vi "Set AO Chan Gain on Fly.vi"(8 "error in (no error)":errorcluster, 9 "Gain Setting":u16(ring) items=["0 dB Gain"=0, "20 dB Gain"=2, "40 dB Gain"=4], 10 "channel":string="AO01") -> (0 "error out":errorcluster)   [LabVIEW 2015]
uses:
  PXI Globals.vi
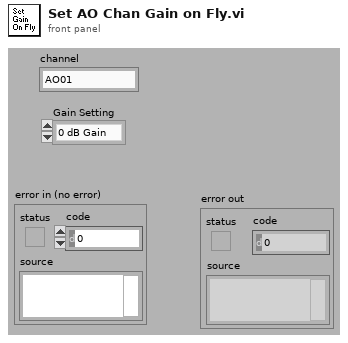
[diagram p1: front panel]
types:
  T1 = typedef "Task Struct.ctl" = cluster{"Task name":string, "Task":refnum<k21>, "Dual-channel task?":bool, "Regenerate?":bool, "Clear?":bool}
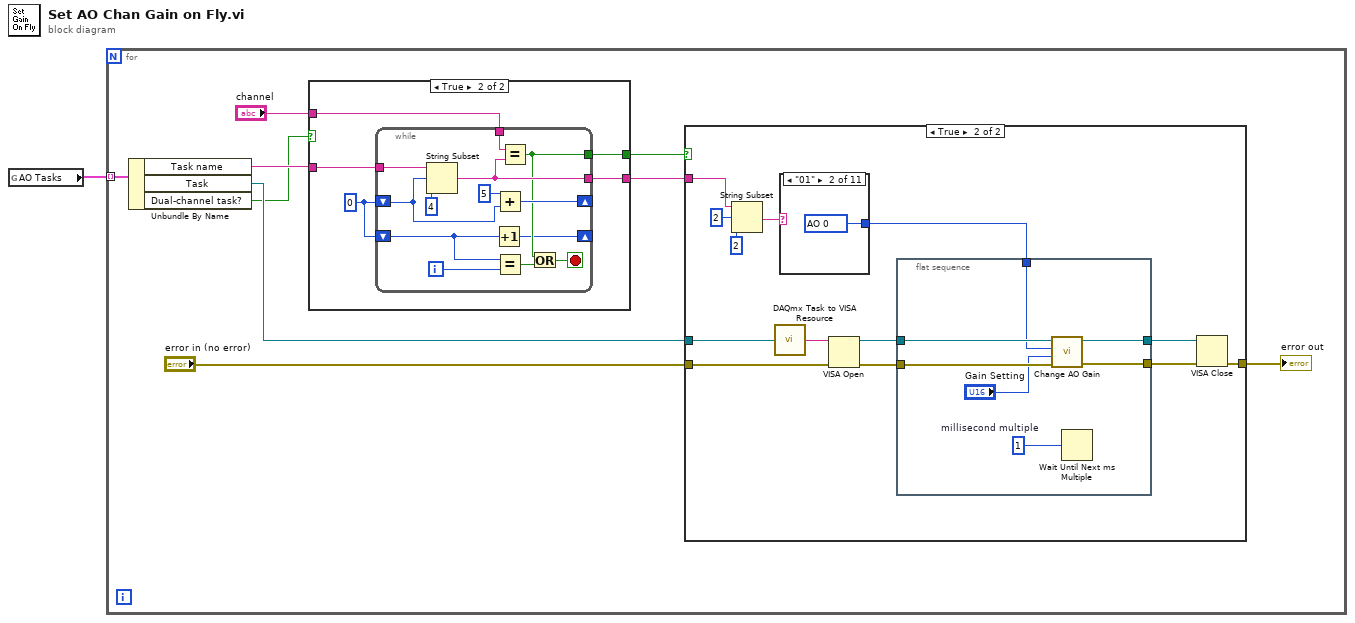
[diagram p0: block diagram]
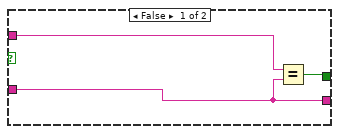
[diagram p2: hidden frame]
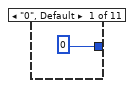
[diagram p4: hidden frame]
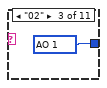
[diagram p5: hidden frame]
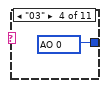
[diagram p6: hidden frame]
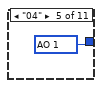
[diagram p7: hidden frame]
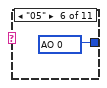
[diagram p8: hidden frame]
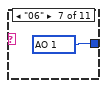
[diagram p9: hidden frame]
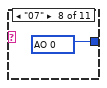
[diagram p10: hidden frame]
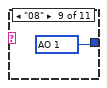
[diagram p11: hidden frame]
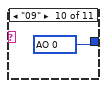
[diagram p12: hidden frame]
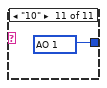
[diagram p13: hidden frame]
diagram:
  n1 = global read "PXI Globals.vi" "AO Tasks"() -> (w1:T1[])
  n2 = for {
    tunnel: w1 -> [w10] mode=indexing
    n3 = Unbundle By Name(w10) -> ("Task name"=w6:string, "Task"=w7:refnum<k21>, "Dual-channel task?"=w5:bool)
    n4 = case shown="True" w5 {
      tunnel: w6 -> [w11 w18]
      tunnel: [w11 w17] -> w4
      tunnel: [w13 w16] -> w3
      tunnel: "channel" -> [w12 w15]
      frame False {
        n5 = Equal?(x=w12, y=w11) -> (x = y?=w13:bool)
      }
      frame True {
        w14 = 0
        n6 = while {
          tunnel: w18 -> [w31]
          tunnel: [w26] -> w17
          shift-right: [w29] -> _
          shift-left: w14 -> [w27]
          tunnel: [w23] -> w16
          tunnel: w15 -> [w25]
          shift-right: [w22] -> _
          shift-left: w14 -> [w20]
          i -> [w19]
          stop <- w24 stop-if-true
          n7 = String Subset(string=w31, offset (0)=w27, length (rest)=4 ("length (rest)")) -> (substring=w26:string)
          n8 = Increment(x=w20) -> (x+1=w22:i32)
          n9 = Add(x=5, y=w27) -> (x+y=w29:i32)
          n10 = Equal?(x=w20, y=w19) -> (x = y?=w21:bool)
          n11 = Equal?(x=w25, y=w26) -> (x = y?=w23:bool)
          n12 = Or(x=w23, y=w21) -> (x .or. y?=w24:bool)
        }
      }
    }
    n13 = case shown="True" w3 {
      tunnel: w7 -> [_ w39]
      tunnel: [w32 w38] -> w9
      tunnel: "error in (no error)" -> [w32 w37]
      tunnel: w4 -> [_ w33]
      frame False {
      }
      frame True {
        n14 = String Subset(string=w33, offset (0)=2, length (rest)=2 ("length (rest)")) -> (substring=w34:string)
        n15 = call "DAQmx Task to VISA Resource.vi"("task out"=w39) -> ("VISAName"=w45:string)  [unwired: 3 in, 1 out]
        n16 = case shown="\"01\"" w34 {
          tunnel: [0 w54 w55 w56 w57 w58 w59 w60 w61 w62 w63] -> w40
          frame "0", Default {
          }
          frame "01" {
            w54 = u16 1536 items=["AO 0"=1536, "AO 1"=1540] ("AO Channel")
          }
          frame "02" {
            w55 = u16 1540 items=["AO 0"=1536, "AO 1"=1540] ("AO Channel")
          }
          frame "03" {
            w56 = u16 1536 items=["AO 0"=1536, "AO 1"=1540] ("AO Channel")
          }
          frame "04" {
            w57 = u16 1540 items=["AO 0"=1536, "AO 1"=1540] ("AO Channel")
          }
          frame "05" {
            w58 = u16 1536 items=["AO 0"=1536, "AO 1"=1540] ("AO Channel")
          }
          frame "06" {
            w59 = u16 1540 items=["AO 0"=1536, "AO 1"=1540] ("AO Channel")
          }
          frame "07" {
            w60 = u16 1536 items=["AO 0"=1536, "AO 1"=1540] ("AO Channel")
          }
          frame "08" {
            w61 = u16 1540 items=["AO 0"=1536, "AO 1"=1540] ("AO Channel")
          }
          frame "09" {
            w62 = u16 1536 items=["AO 0"=1536, "AO 1"=1540] ("AO Channel")
          }
          frame "10" {
            w63 = u16 1540 items=["AO 0"=1536, "AO 1"=1540] ("AO Channel")
          }
        }
        n17 = VISA Open(error in (no error)=w37, VISA resource name=w45) -> (VISA resource name=w41:refnum<visa-resource-name>, error out=w42:errorcluster)  [unwired: 3 in]
        n18 = flat-sequence {
          tunnel: w41 -> [w52]
          tunnel: w42 -> [w51]
          tunnel: [w50] -> w43
          tunnel: [w49] -> w44
          tunnel: w40 -> [w46]
          frame #0 {
            w47 = u32 1  # millisecond multiple
            n19 = call "Change AO Gain.vi"("error in"=w51, "Gain Setting"="Gain Setting", "AO Channel"=w46, "VISA resource name 2"=w52) -> ("error out"=w49:errorcluster, "VISA resource name"=w50:refnum<visa-resource-name>)  [unwired: 4 in]
            n20 = Wait Until Next ms Multiple(millisecond multiple=w47) -> ()  [unwired: 1 out]
          }
        }
        n21 = VISA Close(VISA resource name=w43, error in (no error)=w44) -> (error out=w38:errorcluster)
      }
    }
    "error out" <- w9
  }
